vi "Sigma_MoveAbs.vi"(5 "Direction (+)":bool=TRUE, 7 "Axis (1)":i32=1, 8 "error in (no error)":errorcluster, 9 "Travel (1mm)":dbl=1.0 format="%#_2f", 10 "Travel per Pulse (0.004mm)":dbl=0.004, 11 "VISA resource name":refnum<visa-resource-name>) -> (0 "error out":errorcluster, 3 "VISA resource name out":refnum<visa-resource-name>)   [LabVIEW 2018]
panel:
  out "String Received 3":string
  out "String Received 2":string
  out "String Received":string
  out "결과 문자열":string
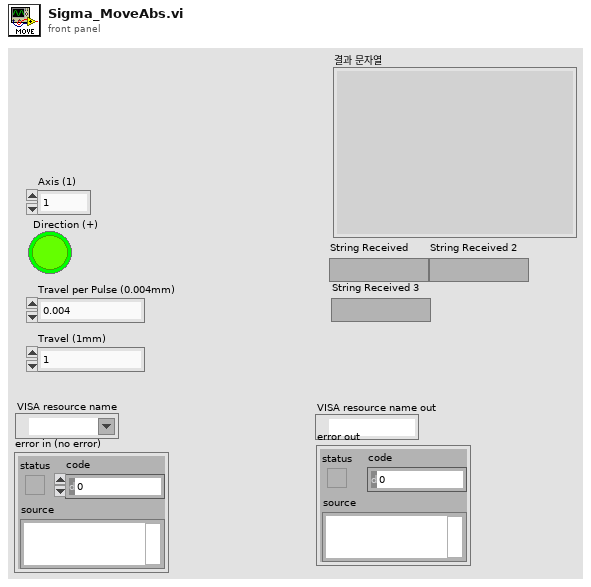
[diagram p1: front panel]
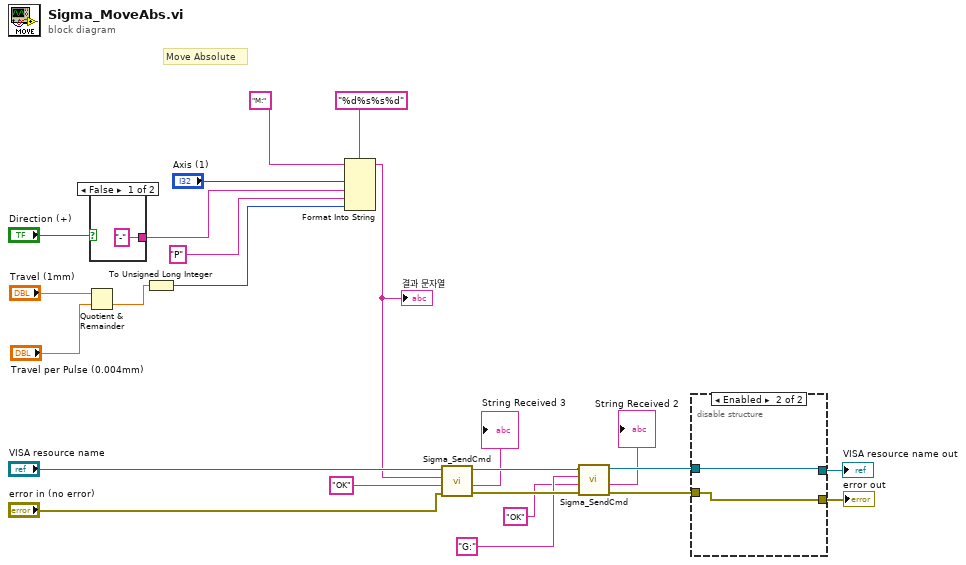
[diagram p0: block diagram]
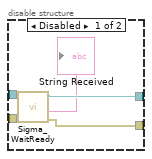
[diagram p2: hidden frame]
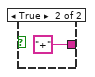
[diagram p3: hidden frame]
diagram:
  # "Move Absolute"
  n1 = Quotient & Remainder(x="Travel (1mm)", y="Travel per Pulse (0.004mm)") -> (floor(x/y)=w16:dbl)  [unwired: 1 out]
  n2 = case shown="False" "Direction (+)" {
    tunnel: ["-" "+"] -> w19
    frame False {
    }
    frame True {
    }
  }
  n3 = To Unsigned Long Integer(number=w16) -> (unsigned 32bit integer=w15:u32)
  n4 = Format Into String(format string="%d%s%s%d", initial string="M:" ("string"), "Axis (1)", w19, "P" ("input 3"), w15) -> (resulting string=w13:string)  [unwired: 1 in, 1 out]
  "결과 문자열" <- w13
  n5 = call "Sigma_SendCmd.vi"("error in (no error)"="error in (no error)", "String to Receive"="OK", "String to Send"=w13, "VISA resource name"="VISA resource name") -> ("error out"=w6:errorcluster, "String Received"=→"String Received 3":string, "VISA resource name out"=w8:refnum<visa-resource-name>)  [unwired: 4 in, 1 out]
  n6 = call "Sigma_SendCmd.vi"("error in (no error)"=w6, "String to Receive"="OK", "String to Send"="G:" ("input 3"), "VISA resource name"=w8) -> ("error out"=w5:errorcluster, "String Received"=→"String Received 2":string, "VISA resource name out"=w7:refnum<visa-resource-name>)  [unwired: 4 in, 1 out]
  n7 = disable-structure shown="Enabled" {
    disable-tunnel: [w31 w32] -> w10
    disable-tunnel: [w30 w33] -> w9
    disable-tunnel: w7 -> [w29 w33]
    disable-tunnel: w5 -> [w28 w32]
    frame Disabled {
      n8 = call "Sigma_WaitReady.vi"("error in (no error)"=w28, "VISA resource name"=w29) -> ("error out"=w31:errorcluster, "String Received"=→"String Received":string, "VISA resource name out"=w30:refnum<visa-resource-name>)  [unwired: 7 in]
    }
    frame Enabled {
    }
  }
  "VISA resource name out" <- w9
  "error out" <- w10
